vi "CAN_Float_Example.vi"() -> ()   [LabVIEW 2016]
panel:
  in  "SubIndex":i32=2 format="%x"
  in  "Index":i32=8194 format="%x"
  in  "CAN Module\nNode ID":i32=3
  out "SDO Float\nResult":sgl format="%#_8g"
  in  "Instrument Type":i32(ring)=2 items=["PPMS", "VersaLab", "DynaCool", "SVSM"]
  in  "Remote":bool=TRUE
  in  "IP Address":string="127.0.0.1"
  # "Instrument Connection"
  # "Float SDO Read"
  # "2002.2 is time since last reset in seconds. This should read a nonzero result."
  # "Node 3 is TCM. Pick a node that is present in your system for this test."
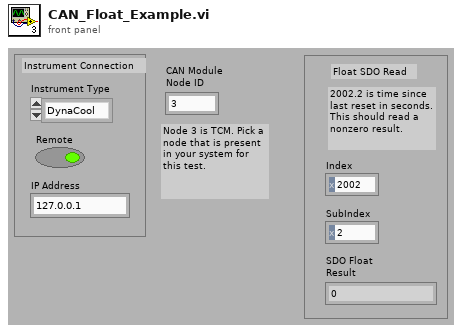
[diagram p1: front panel]
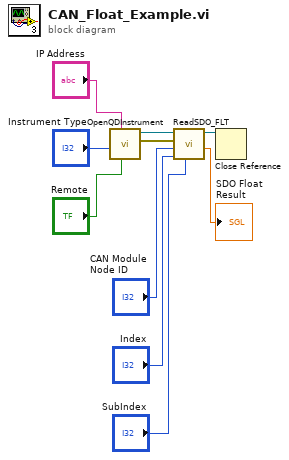
[diagram p0: block diagram]
diagram:
  n1 = call "OpenQDInstrument.vi"("Remote"="Remote", "IP Address"="IP Address", "Instrument Type"="Instrument Type") -> ("error out"=w9:errorcluster, "Instrument Ref"=w10:refnum<k24>)  [unwired: 5 in]
  n2 = call "ReadSDO_FLT.vi"("SubIndex"="SubIndex", "Index"="Index", "nodeID"="CAN Module\nNode ID", "error in (no error)"=w9, "Instrument Ref In"=w10) -> ("SDO Float Result"=→"SDO Float\nResult":sgl, "Instrument Ref Out"=w1:refnum<k24>)  [unwired: 2 in, 1 out]
  n3 = Close Reference(reference=w1) -> ()  [unwired: 1 in, 1 out]
